vi "D2SParser - Private - Helper - Read Long.vi"(8 "error in (no error)":errorcluster, 10 "Position":i64, 11 "D2SParser in":refnum<class "D2SParser.lvclass">) -> (0 "error out":errorcluster, 2 "long":u32, 3 "D2SParser out":refnum<class "D2SParser.lvclass">)   [LabVIEW 2015, in "D2SParser.lvclass"]
uses:
  D2SParser.lvclass
  D2SParser.lvclass/D2SParser.ctl
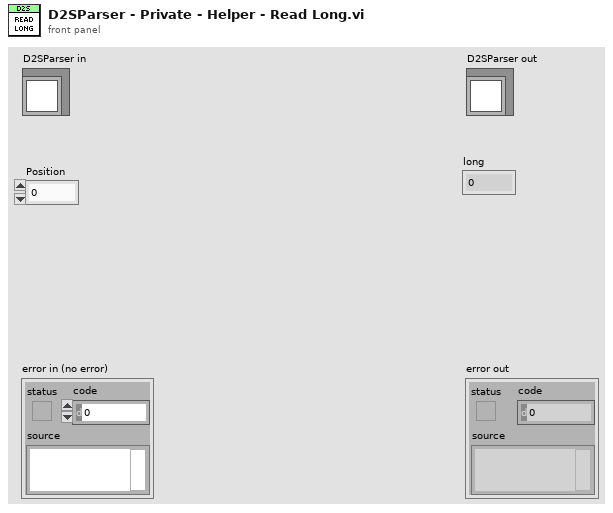
[diagram p1: front panel]
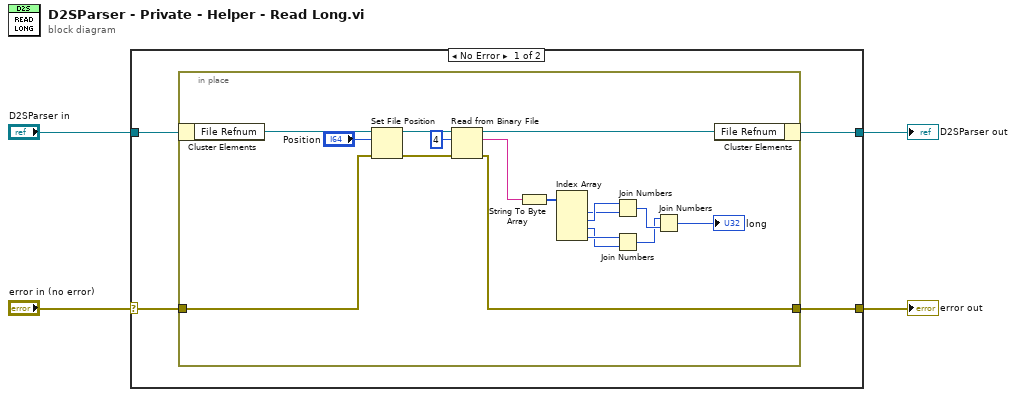
[diagram p0: block diagram]
diagram:
  n1 = case shown="No Error" "error in (no error)" {
    selector: "error in (no error)" -> [w7 w27]
    tunnel: [w6 w27] -> w3
    tunnel: [w5 w26] -> w1
    tunnel: "D2SParser in" -> [w8 w26]
    frame No Error {
      n2 = in-place {
        in-place-border: w7 -> [w20]
        in-place-border: [w17] -> w6
        n3 = in-place-cluster #1(w8) -> ("File Refnum"=w22:refnum<file>)
        n4 = Set File Position(offset (in bytes) (0)="Position", refnum=w22, error in=w20) -> (refnum out=w23:refnum<file>, error out=w24:errorcluster)  [unwired: 1 in]
        n5 = Read from Binary File(8:w24, 10:4 ("count (1)"), 11:w23) -> (0:w17:errorcluster, 2:w16:string, 3:w21:refnum<file>)  [unwired: 3 in, 1 out]
        n6 = String To Byte Array(string=w16) -> (unsigned byte array=w18:u8[])
        n7 = Index Array(array=w18) -> (element #1=w14:u8, element #2=w15:u8, element #3=w12:u8, element #4=w13:u8)  [unwired: 4 in]
        n8 = Join Numbers(hi=w15, lo=w14) -> ((hi.lo)=w11:u16)
        n9 = Join Numbers(hi=w13, lo=w12) -> ((hi.lo)=w10:u16)
        n10 = Join Numbers(hi=w10, lo=w11) -> ((hi.lo)=→"long":u32)
        n11 = in-place-cluster #1("File Refnum"=w21) -> (w5:refnum<class "D2SParser.lvclass">)
      }
    }
    frame Error {
    }
  }
  "error out" <- w3
  "D2SParser out" <- w1
